vi "_Yt05_Rendezvous.vi"(11 "YTESTER测试数据":T1 caption="不要修改！") -> (3 "YTESTER结论":T2)   [LabVIEW 2017]
doc: "VIClassID=YT_SSTEPFLAG_RENDEZVOUS\nVIDescription=这是一个集合步骤，用于多DUT测试中等待同步。"
uses:
  YtCommon.lvlibp/yt`Step StepBaseInput.ctl
  YtCommon.lvlibp/yt`Step StepResult.ctl
  YtCommon.lvlibp/yt`Step TestData.ctl
  YtCommon.lvlibp/yt`Step System Queue.ctl
  Step`s VIs/YYLLGeneric/variable_W.ctl
  YtCommon.lvlibp/yt`Data-Ytester Type Data.ctl
  eb6acbc6-6d25-4169-8be2-d3db0eea80d1.vi
  3d7e4338-b3ba-4f78-9b53-bb35a90ad2a8.vi
  c6f87483-778a-4cd7-a727-6f77e22eec7d.vi
  e4cbf99c-6f59-48e8-a6b4-cf35277f6964.vi
  <vilib>/Utility/error.llb/Clear Errors.vi
  YtCommon.lvlibp/yt`varSystemlib IO Read Variable.vi
  YtCommon.lvlibp
panel:
  in  "YTESTER开放参数":T4={"YTESTER_BaseInput"={"isTest"=TRUE, "isSkip"=FALSE, "StepName"="集合", "OnPass"=enum."Next", "OnFail"=enum."Terminate", "ReTestNumber"=0.0}, "集合名称（空使用StepName）"="", "集合达成数量（<0是自动）"=-1, "超时s"=-1.0}
  # "集合！"
  # "#yyll 首先这个必须是重入VI"
  # "YT_SSTEPFLAG_RENDEZVOUS"
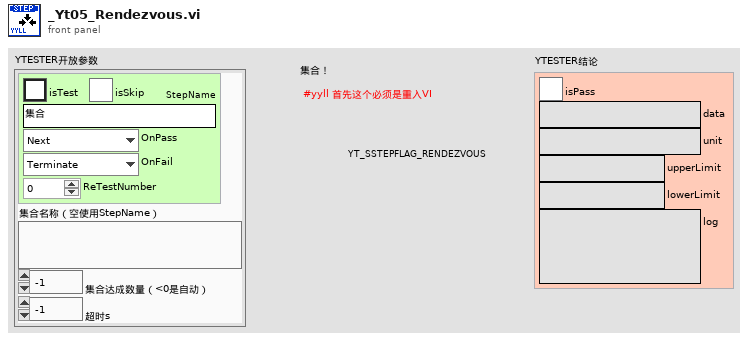
[diagram p1: front panel]
types:
  T1 = typedef "YtCommon.lvlibp/yt`Step TestData.ctl" = cluster{"Socket(From1)":i32, "SN":refnum<notifier>, "StopFlagRef":refnum<notifier>, "YT System Queue":refnum<queue>}
  T2 = typedef "YtCommon.lvlibp/yt`Step StepResult.ctl" = cluster{"isPass":bool, "data":string, "unit":string, "upperLimit":string, "lowerLimit":string, "log":string}
  T3 = typedef "YtCommon.lvlibp/yt`Step StepBaseInput.ctl" = cluster{"isTest":bool, "isSkip":bool, "StepName":string, "OnPass":enum16{"Next", "ToOVER", "Terminate"}, "OnFail":enum16{"Next", "ToOVER", "Terminate"}, "ReTestNumber":dbl}
  T4 = cluster{"YTESTER_BaseInput":T3, "集合名称（空使用StepName）":string, "集合达成数量（<0是自动）":i32, "超时s":dbl}
  T5 = typedef "YtCommon.lvlibp/yt`Step System Queue.ctl" = cluster{"Socket(From0)":i32, "Cmd":string, "Data":variant}
  T6 = typedef "variable_W.ctl" = cluster{"YT_TYPE":T7, "TypeData":string[], "Tips":string}
  T7 = typedef "YtCommon.lvlibp/yt`Data-Ytester Type Data.ctl" = enum16{"NULL", "NUM", "BOOL", "TXT", "ENUM", "TIME", "PATH", "VISA", "COMBO", "ColorBox", "RadioBtn", "Array_NUM", "Array_BOOL", "Array_TXT", "Array_ENUM", "Array_PATH", "Array_COMBO"}
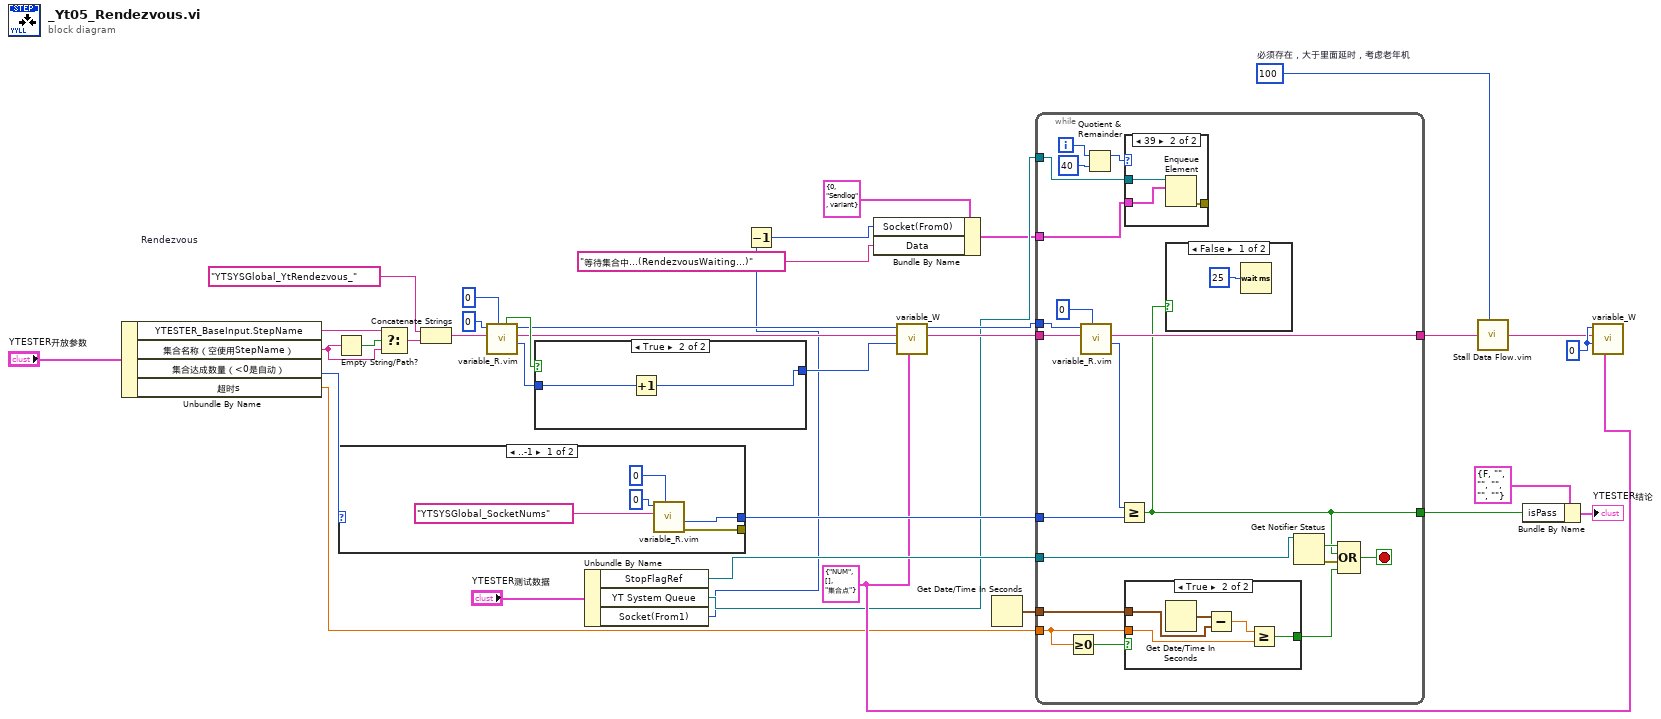
[diagram p0: block diagram]
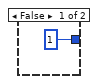
[diagram p5: hidden frame]
diagram:
  w11 = u32 100  # 必须存在，大于里面延时，考虑老年机
  w14 = 0 ("函数池名称 in")
  w13 = T6 {"YT_TYPE"=enum."NUM", "TypeData"=[], "Tips"="集合点"} ("附加的Information")
  w27 = "YTSYSGlobal_YtRendezvous_"  # Rendezvous
  n1 = Unbundle By Name("YTESTER开放参数") -> ("YTESTER_BaseInput.StepName"=w31:string, "集合名称（空使用StepName）"=w33:string, "集合达成数量（<0是自动）"=w30:i32, "超时s"=w4:dbl)
  n2 = Empty String/Path?(string/path=w33) -> (empty?=w34:bool)
  n3 = case shown="..-1" w30 {
    selector: w30 -> [_ w42]
    tunnel: [w38 w42] -> w29
    tunnel: [w37 _] -> _
    frame ..-1 {
      n4 = call "variable_R.vim"("type"=0 ("集合达成数量(<0是自动)"), "待获取变量名称"="YTSYSGlobal_SocketNums", "函数池名称"=0) -> ("error out"=w37:errorcluster, "value"=w38:i32)  [unwired: 4 in, 3 out]
    }
    frame 0.. {
    }
  }
  n5 = Select(t=w31, s=w34, f=w33) -> (s? t:f=w32:string)
  n6 = Concatenate Strings(w27, w32) -> (w28:string)
  n7 = call "variable_R.vim"("type"=0 ("函数池名称"), "待获取变量名称"=w28, "函数池名称"=0) -> ("value"=w22:i32, "待获取变量名out"=w20:string, "函数池名称out"=w21:i32, "found?"=w23:bool)  [unwired: 4 in, 1 out]
  n8 = case shown="True" w23 {
    tunnel: w22 -> [_ w45]
    tunnel: [1 w44] -> w19
    frame False {
    }
    frame True {
      n9 = Increment(x=w45) -> (x+1=w44:i32)
    }
  }
  n10 = Unbundle By Name("YTESTER测试数据") -> ("StopFlagRef"=w18:refnum<notifier>, "YT System Queue"=w10:refnum<queue>, "Socket(From1)"=w6:i32)
  n11 = Decrement(x=w6) -> (x-1=w5:i32)
  n12 = Bundle By Name(cluster=T5 {"Socket(From0)"=0, "Cmd"="Sendlog", "Data"=variant} ("element"), "Socket(From0)"=w5, "Data"="等待集合中...(RendezvousWaiting...)" ("Tips")) -> (w8:T5)
  n13 = call "variable_W.vi"("附加的Information"=w13, "待写入池的输入控件"=w19, "待写入池变量名称"=w20, "函数池名称 in"=w21) -> ("待写入池变量名称out"=w16:string, "函数池名称 out"=w17:i32)  [unwired: 5 in, 1 out]
  n14 = Get Date/Time In Seconds() -> (seconds since 1Jan1904=w3:timestamp)
  n15 = while {
    tunnel: w18 -> [w65]
    tunnel: w17 -> [w64]
    tunnel: w16 -> [w63]
    tunnel: w29 -> [w60]
    tunnel: [w57] -> w15
    tunnel: w10 -> [w52]
    tunnel: w8 -> [w51]
    tunnel: w4 -> [w48]
    tunnel: w3 -> [w49]
    tunnel: [w46] -> w1
    i -> [w55]
    stop <- w58 stop-if-true
    n16 = Greater Or Equal To 0?(x=w48) -> (x >= 0?=w50:bool)
    n17 = call "variable_R.vim"("type"=0 ("函数池名称"), "待获取变量名称"=w63, "函数池名称"=w64) -> ("value"=w61:i32, "待获取变量名out"=w57:string)  [unwired: 4 in, 3 out]
    n18 = Quotient & Remainder(x=w55, y=40) -> (x-y*floor(x/y)=w53:i32)  [unwired: 1 out]
    n19 = Greater Or Equal?(x=w61, y=w60) -> (x >= y?=w46:bool)
    n20 = case shown="39" w53 {
      tunnel: w52 -> [_ w73]
      tunnel: w51 -> [_ w72]
      tunnel: [_ w71] -> _
      frame 0, Default {
      }
      frame 39 {
        n21 = Enqueue Element(queue=w73, element=w72) -> (error out=w71:errorcluster)  [unwired: 2 in, 2 out]
      }
    }
    n22 = case shown="True" w50 {
      tunnel: w49 -> [_ w69]
      tunnel: w48 -> [_ w67]
      tunnel: [_ w66] -> w47
      frame False {
      }
      frame True {
        n23 = Get Date/Time In Seconds() -> (seconds since 1Jan1904=w70:timestamp)
        n24 = Subtract(x=w70, y=w69) -> (x-y=w68:dbl)
        n25 = Greater Or Equal?(x=w68, y=w67) -> (x >= y?=w66:bool)
      }
    }
    n26 = case shown="False" w46 {
      frame False {
        n27 = Wait (ms)(milliseconds to wait=u32 25) -> ()  [unwired: 1 out]
      }
      frame True {
      }
    }
    n28 = Get Notifier Status(notifier=w65) -> (current notification=w59:bool, error out=w56:errorcluster)  [unwired: 1 in, 3 out]
    n29 = Compound Arithmetic op=OR(w59, w46, w56, w47) -> (w58:bool)
  }
  n30 = call "Stall Data Flow.vim"("value in"=w15, "milliseconds to wait"=w11) -> ("value out"=w12:string)  [unwired: 1 out]
  n31 = Bundle By Name(cluster=T2 {"isPass"=FALSE, "data"="", "unit"="", "upperLimit"="", "lowerLimit"="", "log"=""} ("Result"), "isPass"=w1) -> (→"YTESTER结论":T2)
  n32 = call "variable_W.vi"("附加的Information"=w13, "待写入池的输入控件"=w14, "待写入池变量名称"=w12, "函数池名称 in"=w14) -> ()  [unwired: 5 in, 3 out]
